vi "UI - Initiate Connection.vi"(8 "error in (no error)":errorcluster, 10 "Controller Address":string, 11 "Message Queue":refnum<queue>) -> (0 "error out":errorcluster, 1 "Connected?":bool)   [LabVIEW 2013]
uses:
  Message Queue/Message Cluster.ctl
  controls/Raw Values.ctl
  controls/FPGA State.ctl
  controls/Controller Calcs.ctl
  controls/Observer Calcs.ctl
  controls/Other Calcs.ctl
  controls/Variable References.ctl
  Globals/Global - Configuration Options.vi
  Globals/Global - UI Stream and Variable Connections.vi
  Message Queue/Message Queue.lvlib
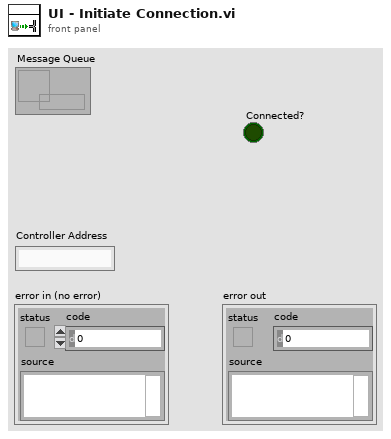
[diagram p1: front panel]
types:
  T1 = typedef "Other Calcs.ctl" = cluster{"k_1 (1/s)":fxp<+/-,20,7>, "k_2 (1/s)":fxp<+/-,20,7>, "Frr (N/s)":fxp<+/-,20,7>, "xrr (mm/s)":fxp<+/-,20,14>}
  T2 = typedef "Observer Calcs.ctl" = cluster{"bo (kg/s)":fxp<+/-,20,7>, "kso (N/m)":fxp<+/-,20,7>, "kiso (N/m)":fxp<+/-,20,7>}
  T3 = typedef "Controller Calcs.ctl" = cluster{"ba (kg/s)":fxp<+/-,20,7>, "ksa (N/m)":fxp<+/-,20,7>, "kisa (N/m)":fxp<+/-,20,7>, "k_backemf (Vs/m)":fxp<+/-,20,14>}
  T4 = typedef "FPGA State.ctl" = enum16{"Safe State", "Manual", "Control (PID)"}
  T5 = typedef "Raw Values.ctl" = cluster{"Channel 0":fxp<+/-,20,7>, "Channel 1":fxp<+/-,20,7>, "Channel 2":fxp<+/-,20,7>, "Channel 3":fxp<+/-,20,14>}
  T6 = typedef "Message Queue.lvlib/Message Cluster.ctl" = cluster{"Message":string, "Message Data":variant}
  T7 = typedef "Variable References.ctl" = cluster{"CPU Usage":refnum<k21>, "Contiguous Memory":refnum<k21>, "Input Values":refnum<k21>, "Output Values":refnum<k21>, "FPGA Mode":refnum<k21>, "Actual Loop Period":refnum<k21>, "Controller Calcs":refnum<k21>, "Observer Calcs":refnum<k21>, "Other Calcs":refnum<k21>}
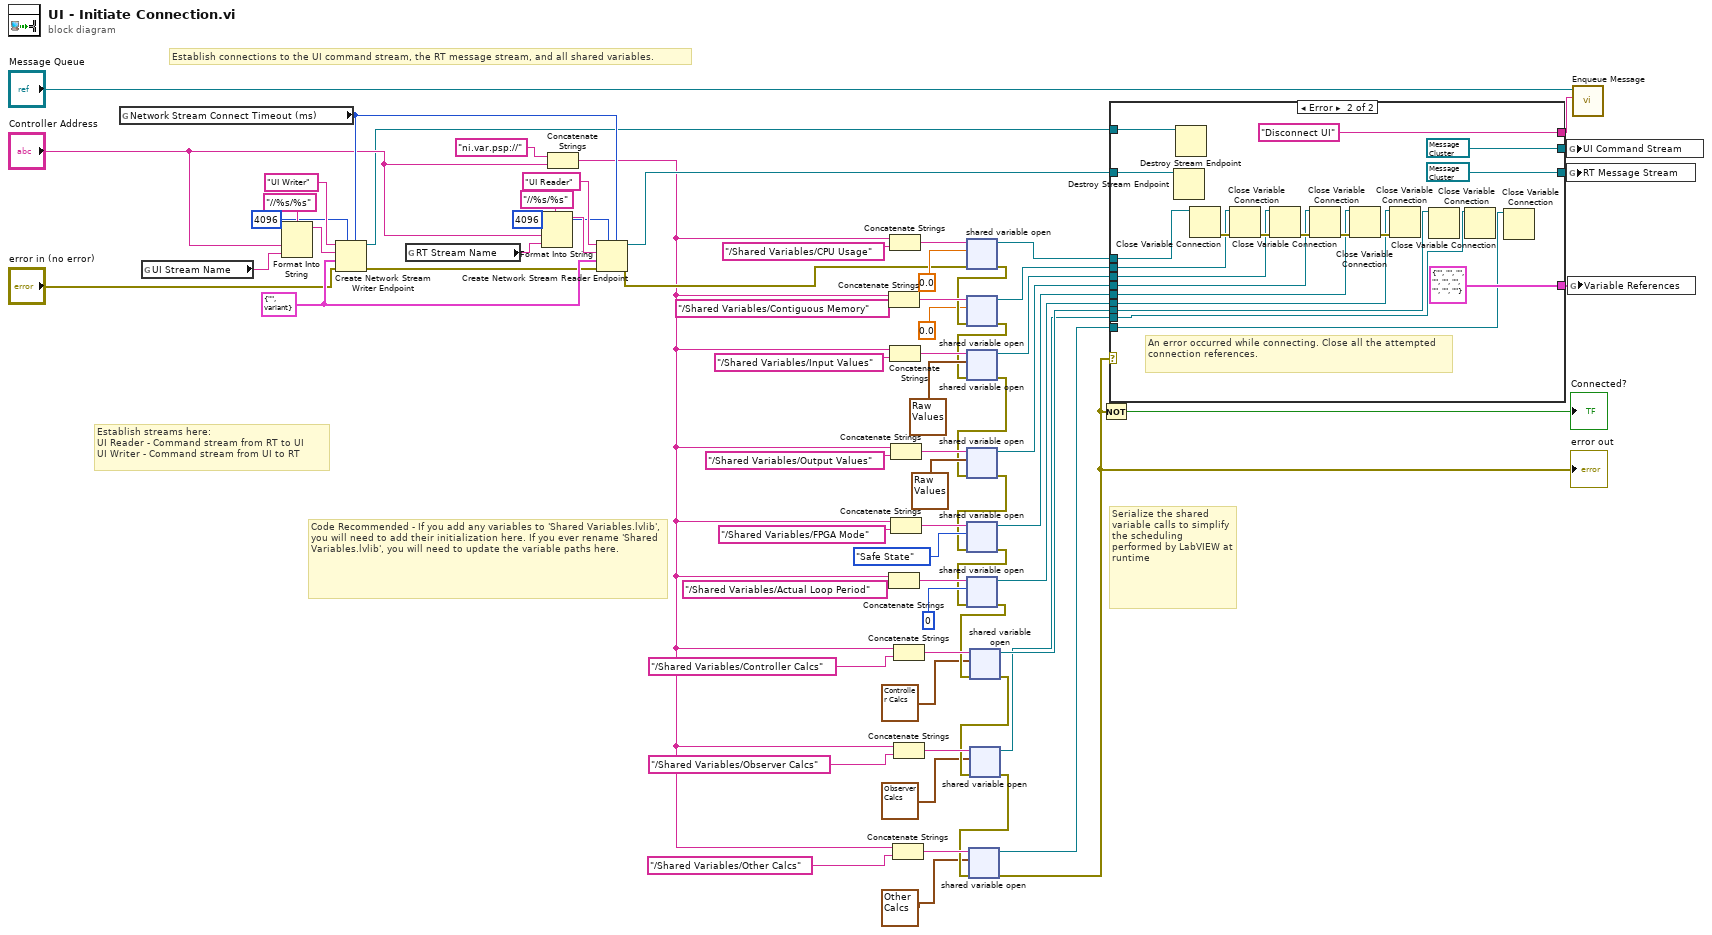
[diagram p0: block diagram]
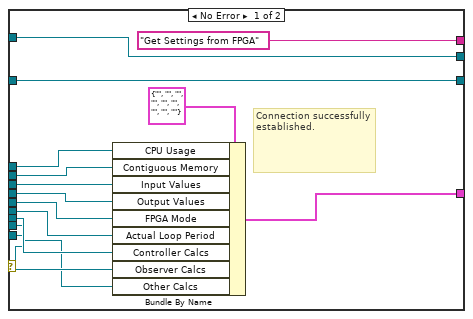
[diagram p2: hidden frame]
diagram:
  w62 = T6 {"Message"="", "Message Data"=variant} ("Message Cluster")
  # "Establish connections to the UI command stream, the RT message stream, and all shared variables."
  # "Code Recommended - If you add any variables to 'Shared Variables.lvlib', you will need to add their initialization here. If you ever rename 'Shared Variables.lvlib', you will need to update the variable paths here."
  # "Establish streams here:\nUI Reader - Command stream from RT to UI\nUI Writer - Command stream from UI to RT"
  # "Serialize the shared variable calls to simplify the scheduling performed by LabVIEW at runtime"
  n1 = global read "Global - Configuration Options.vi" "Network Stream Connect Timeout (ms)"() -> (w61:i32)
  n2 = global read "Global - Configuration Options.vi" "UI Stream Name"() -> (w69:string)
  n3 = Format Into String(format string="//%s/%s", "Controller Address", w69) -> (resulting string=w68:string)  [unwired: 2 in, 1 out]
  n4 = Create Network Stream Writer Endpoint(5:w61, 7:4096 ("writer buffer size"), 8:"error in (no error)", 9:w62, 10:w68, 11:"UI Writer" ("writer name")) -> (0:w22:errorcluster, 3:w30:refnum<k21>)  [unwired: 1 in]
  n5 = global read "Global - Configuration Options.vi" "RT Stream Name"() -> (w66:string)
  n6 = Format Into String(format string="//%s/%s", "Controller Address", w66) -> (resulting string=w65:string)  [unwired: 2 in, 1 out]
  n7 = Concatenate Strings("ni.var.psp://", "Controller Address") -> (w3:string)
  n8 = Create Network Stream Reader Endpoint(5:w61, 7:4096 ("reader buffer size"), 8:w22, 9:w62, 10:w65, 11:"UI Reader" ("reader name")) -> (0:w21:errorcluster, 3:w29:refnum<k21>)  [unwired: 1 in]
  n9 = Concatenate Strings(w3, "/Shared Variables/Contiguous Memory") -> (w54:string)
  n10 = Concatenate Strings(w3, "/Shared Variables/Actual Loop Period") -> (w46:string)
  n11 = Concatenate Strings(w3, "/Shared Variables/CPU Usage") -> (w57:string)
  n12 = Concatenate Strings(w3, "/Shared Variables/Input Values") -> (w52:string)
  n13 = Concatenate Strings(w3, "/Shared Variables/Output Values") -> (w50:string)
  n14 = Concatenate Strings(w3, "/Shared Variables/FPGA Mode") -> (w49:string)
  n15 = Concatenate Strings(w3, "/Shared Variables/Other Calcs") -> (w7:string)
  n16 = Concatenate Strings(w3, "/Shared Variables/Controller Calcs") -> (w17:string)
  n17 = Concatenate Strings(w3, "/Shared Variables/Observer Calcs") -> (w12:string)
  n18 = shared-variable-open(w57, w21, 0.0) -> (w36:refnum<k21>, w41:errorcluster)  [unwired: 1 in]
  n19 = shared-variable-open(w54, w41, 0.0) -> (w35:refnum<k21>, w40:errorcluster)  [unwired: 1 in]
  n20 = shared-variable-open(w52, w40, T5 {"Channel 0"=0.0, "Channel 1"=0.0, "Channel 2"=0.0, "Channel 3"=0.0}) -> (w34:refnum<k21>, w39:errorcluster)  [unwired: 1 in]
  n21 = shared-variable-open(w50, w39, T5 {"Channel 0"=0.0, "Channel 1"=0.0, "Channel 2"=0.0, "Channel 3"=0.0}) -> (w33:refnum<k21>, w38:errorcluster)  [unwired: 1 in]
  n22 = shared-variable-open(w49, w38, FPGA_State."Safe State" ("FPGA State")) -> (w32:refnum<k21>, w37:errorcluster)  [unwired: 1 in]
  n23 = shared-variable-open(w46, w37, u32 0) -> (w31:refnum<k21>, w15:errorcluster)  [unwired: 1 in]
  n24 = shared-variable-open(w17, w15, T3 {"ba (kg/s)"=0.0, "ksa (N/m)"=0.0, "kisa (N/m)"=0.0, "k_backemf (Vs/m)"=0.0} ("Controller Calculations")) -> (w14:refnum<k21>, w10:errorcluster)  [unwired: 1 in]
  n25 = shared-variable-open(w12, w10, T2 {"bo (kg/s)"=0.0, "kso (N/m)"=0.0, "kiso (N/m)"=0.0} ("Observer Calculations")) -> (w9:refnum<k21>, w5:errorcluster)  [unwired: 1 in]
  n26 = shared-variable-open(w7, w5, T1 {"k_1 (1/s)"=0.0, "k_2 (1/s)"=0.0, "Frr (N/s)"=0.0, "xrr (mm/s)"=0.0} ("Other Calcs")) -> (w1:refnum<k21>, w4:errorcluster)  [unwired: 1 in]
  "error out" <- w4
  n27 = Not(x=w4) -> (.not. x?=→"Connected?":bool)
  n28 = case shown="Error" w4 {
    tunnel: w36 -> [w84 w98]
    tunnel: w35 -> [w83 w93]
    tunnel: w34 -> [w82 w94]
    tunnel: w33 -> [w81 w95]
    tunnel: w32 -> [w80 w96]
    tunnel: w31 -> [w79 w97]
    tunnel: w30 -> [w75 w104]
    tunnel: w29 -> [w77 w105]
    tunnel: [w78 T7 {"CPU Usage"="", "Contiguous Memory"="", "Input Values"="", "Output Values"="", "FPGA Mode"="", "Actual Loop Period"="", "Controller Calcs"="", "Observer Calcs"="", "Other Calcs"=""} ("Variable References")] -> w28
    tunnel: [w77 refnum<k21> refnum] -> w27
    tunnel: [w75 refnum<k21> refnum] -> w26
    tunnel: ["Get Settings from FPGA" "Disconnect UI"] -> w24
    tunnel: w14 -> [w74 w88]
    tunnel: w9 -> [w73 w87]
    tunnel: w1 -> [w72 w86]
    frame No Error {
      # "Connection successfully established."
      n29 = Bundle By Name(cluster=T7 {"CPU Usage"="", "Contiguous Memory"="", "Input Values"="", "Output Values"="", "FPGA Mode"="", "Actual Loop Period"="", "Controller Calcs"="", "Observer Calcs"="", "Other Calcs"=""} ("Variable References"), "CPU Usage"=w84, "Contiguous Memory"=w83, "Input Values"=w82, "Output Values"=w81, "FPGA Mode"=w80, "Actual Loop Period"=w79, "Controller Calcs"=w74, "Observer Calcs"=w73, "Other Calcs"=w72) -> (w78:T7)
    }
    frame Error {
      # "An error occurred while connecting. Close all the attempted connection references."
      n30 = Destroy Stream Endpoint(11:w105) -> ()  [unwired: 1 in, 1 out]
      n31 = Destroy Stream Endpoint(11:w104) -> ()  [unwired: 1 in, 1 out]
      n32 = Close Variable Connection(11:w98) -> (0:w99:errorcluster)  [unwired: 1 in]
      n33 = Close Variable Connection(8:w99, 11:w93) -> (0:w100:errorcluster)
      n34 = Close Variable Connection(8:w100, 11:w94) -> (0:w101:errorcluster)
      n35 = Close Variable Connection(8:w101, 11:w95) -> (0:w102:errorcluster)
      n36 = Close Variable Connection(8:w102, 11:w96) -> (0:w103:errorcluster)
      n37 = Close Variable Connection(8:w103, 11:w97) -> ()  [unwired: 1 out]
      n38 = Close Variable Connection(11:w88) -> ()  [unwired: 1 in, 1 out]
      n39 = Close Variable Connection(11:w87) -> ()  [unwired: 1 in, 1 out]
      n40 = Close Variable Connection(11:w86) -> ()  [unwired: 1 in, 1 out]
    }
  }
  n41 = global write "Global - UI Stream and Variable Connections.vi" "UI Command Stream"(w26) -> ()
  n42 = global write "Global - UI Stream and Variable Connections.vi" "RT Message Stream"(w27) -> ()
  n43 = global write "Global - UI Stream and Variable Connections.vi" "Variable References"(w28) -> ()
  n44 = call "Enqueue Message.vi"("Message"=w24, "Message Queue"="Message Queue") -> ()  [unwired: 8 in, 2 out]
